vi "PDP Setpoint= Message.vi"(0 "Setpoint":dbl format="%.3f") -> ()   [LabVIEW 2009]
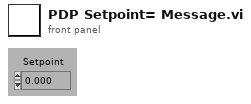
[diagram p1: front panel]
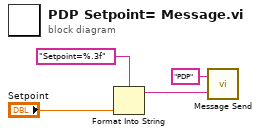
[diagram p0: block diagram]
diagram:
  n1 = Format Into String(format string="Setpoint=%.3f" ("Format String"), "Setpoint") -> (resulting string=w1:string)  [unwired: 2 in, 1 out]
  n2 = call "Message Send.vi"("Message"=w1, "Destination"="PDP") -> ()
